vi "SSI PR Pump Test.vi"() -> ()   [LabVIEW 2018]
uses:
  SSI PR Settings Cluster.ctl
panel:
  out "error out":errorcluster
  in  "error in (no error)":errorcluster
  out "SSI PR Settings Out":T1={"VISA resource name"="", "Simulated?"=TRUE}
  in  "SSI PR Settings In":T1={"VISA resource name"="", "Simulated?"=TRUE}
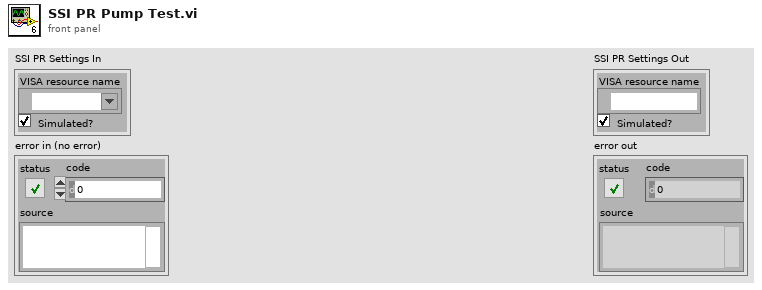
[diagram p1: front panel]
types:
  T1 = typedef "SSI PR Settings Cluster.ctl" = cluster{"VISA resource name":refnum<visa-resource-name>, "Simulated?":bool}
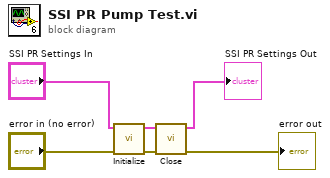
[diagram p0: block diagram]
diagram:
  n1 = call "Initialize.vi"("error in (no error)"="error in (no error)", "SSI PR Settings In"="SSI PR Settings In") -> ("error out"=w2:errorcluster, "SSI PR Settings Out"=w4:T1)  [unwired: 6 in, 2 out]
  n2 = call "Close.vi"("error in (no error)"=w2, "SSI PR Settings In"=w4) -> ("error out"=→"error out":errorcluster, "SSI PR Settings Out"=→"SSI PR Settings Out":T1)  [unwired: 8 in]
